vi "SRV_Update All Motors Config Array.vi"(0 "All Motor Control Config":T1[](array[typedef]) {"Release Cmds"."Motor Control Commands Array"."Value" format="%02x"; "Release Cmds"."Motor Control Commands Array"."Register" format="%02x"; "Release Cmds"."Motor Control Commands Array"."I2C Address" format="%02x"; "Press Cmds"."Motor Control Commands Array"."Value" format="%02x"; "Press Cmds"."Motor Control Commands Array"."Register" format="%02x"; "Press Cmds"."Motor Control Commands Array"."I2C Address" format="%02x"}, 5 "Motor Control Config GUI":T6={"Motor Control Button Index 0"={"Button Name"="Button xx", "Button Label"="", "Motor Type"=enum."Servo", "Press Cmds"={"Motor Control Commands Array"=[]}, "Release Cmds"={"Motor Control Commands Array"=[]}, "Icon"=0}, "Motor Control Button Index 1"={"Button Name"="Button xx", "Button Label"="", "Motor Type"=enum."Servo", "Press Cmds"={"Motor Control Commands Array"=[]}, "Release Cmds"={"Motor Control Commands Array"=[]}, "Icon"=0}, "Motor Control Button Index 2"={"Button Name"="Button xx", "Button Label"="", "Motor Type"=enum."Servo", "Press Cmds"={"Motor Control Commands Array"=[]}, "Release Cmds"={"Motor Control Commands Array"=[]}, "Icon"=0}} {"Motor Control Button Index 2"."Release Cmds"."Motor Control Commands Array"."Value" format="%02x"; "Motor Control Button Index 2"."Release Cmds"."Motor Control Commands Array"."Register" format="%02x"; "Motor Control Button Index 2"."Release Cmds"."Motor Control Commands Array"."I2C Address" format="%02x"; "Motor Control Button Index 2"."Press Cmds"."Motor Control Commands Array"."Value" format="%02x"; "Motor Control Button Index 2"."Press Cmds"."Motor Control Commands Array"."Register" format="%02x"; "Motor Control Button Index 2"."Press Cmds"."Motor Control Commands Array"."I2C Address" format="%02x"; "Motor Control Button Index 1"."Release Cmds"."Motor Control Commands Array"."Value" format="%02x"; "Motor Control Button Index 1"."Release Cmds"."Motor Control Commands Array"."Register" format="%02x"; "Motor Control Button Index 1"."Release Cmds"."Motor Control Commands Array"."I2C Address" format="%02x"; "Motor Control Button Index 1"."Press Cmds"."Motor Control Commands Array"."Value" format="%02x"; "Motor Control Button Index 1"."Press Cmds"."Motor Control Commands Array"."Register" format="%02x"; "Motor Control Button Index 1"."Press Cmds"."Motor Control Commands Array"."I2C Address" format="%02x"; "Motor Control Button Index 0"."Release Cmds"."Motor Control Commands Array"."Value" format="%02x"; "Motor Control Button Index 0"."Release Cmds"."Motor Control Commands Array"."Register" format="%02x"; "Motor Control Button Index 0"."Release Cmds"."Motor Control Commands Array"."I2C Address" format="%02x"; "Motor Control Button Index 0"."Press Cmds"."Motor Control Commands Array"."Value" format="%02x"; "Motor Control Button Index 0"."Press Cmds"."Motor Control Commands Array"."Register" format="%02x"; "Motor Control Button Index 0"."Press Cmds"."Motor Control Commands Array"."I2C Address" format="%02x"}, 12 "Row Start Index":i32) -> (4 "All Motor Control Config out":T1[](array[typedef]) {"Release Cmds"."Motor Control Commands Array"."Value" format="%02x"; "Release Cmds"."Motor Control Commands Array"."Register" format="%02x"; "Release Cmds"."Motor Control Commands Array"."I2C Address" format="%02x"; "Press Cmds"."Motor Control Commands Array"."Value" format="%02x"; "Press Cmds"."Motor Control Commands Array"."Register" format="%02x"; "Press Cmds"."Motor Control Commands Array"."I2C Address" format="%02x"})   [LabVIEW 2014]
doc: "Author: Mike Schultz (LogicPD, Inc)"
uses:
  SRV_Motor Control Button Config.ctl
  SRV_Motor Legos-Servo.ctl
  SRV_Motor Control Commands Cluster.ctl
  SRV_Motor Control Command Config.ctl
  SRV_Motor Control Button Icons_FALSE.ctl
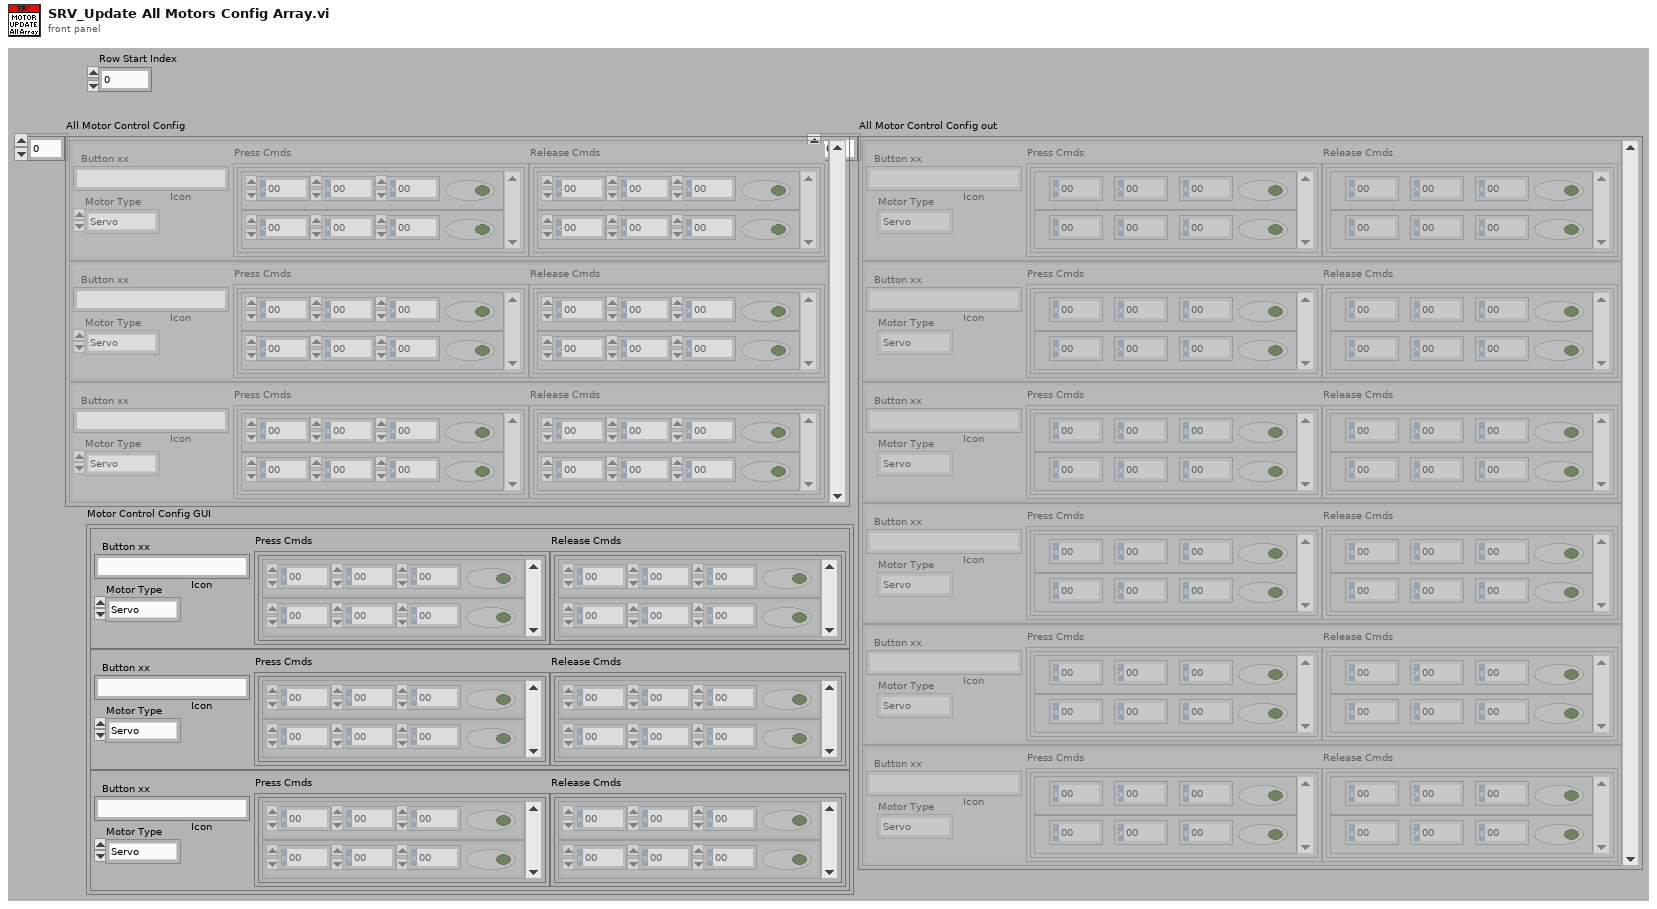
[diagram p1: front panel]
types:
  T1 = typedef "SRV_Motor Control Button Config.ctl" = cluster{"Button Name":string, "Button Label":string, "Motor Type":T2, "Press Cmds":T3, "Release Cmds":T3, "Icon":T5}
  T2 = typedef "SRV_Motor Legos-Servo.ctl" = enum16{"Servo", "Legos", "Shared Var"}
  T3 = typedef "SRV_Motor Control Commands Cluster.ctl" = cluster{"Motor Control Commands Array":T4[]}
  T4 = typedef "SRV_Motor Control Command Config.ctl" = cluster{"I2C Address":u8, "Register":u8, "Value":u8, "Active":bool}
  T5 = typedef "SRV_Motor Control Button Icons_FALSE.ctl" = u16
  T6 = cluster{"Motor Control Button Index 0":T1, "Motor Control Button Index 1":T1, "Motor Control Button Index 2":T1}
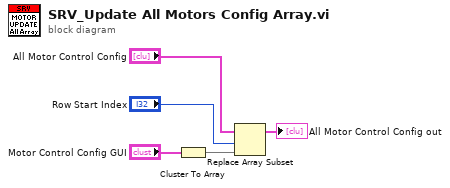
[diagram p0: block diagram]
diagram:
  n1 = Cluster To Array(cluster="Motor Control Config GUI") -> (array=w2:T1[])
  n2 = Replace Array Subset(array="All Motor Control Config", new element=w2, index="Row Start Index") -> (→"All Motor Control Config out":T1[])
